vi "_Parse ACLR NR Limit Check Result.vi"(8 "error in (no error)":errorcluster, 10 "Input String":string, 11 "VISA resource name":refnum<visa-resource-name>) -> (0 "error out":errorcluster, 1 "ACLR Limit Check Results":T1, 2 "Reliability":i32, 3 "VISA resource name out":refnum<visa-resource-name>)   [LabVIEW 2020, in "Rohde&Schwarz CMWXP NR FR1 Measurement.lvlib"]
uses:
  <instrlib>/Rohde&Schwarz CMWXP NR FR1 Measurement/Rohde&Schwarz CMWXP NR FR1 Measurement.lvlib
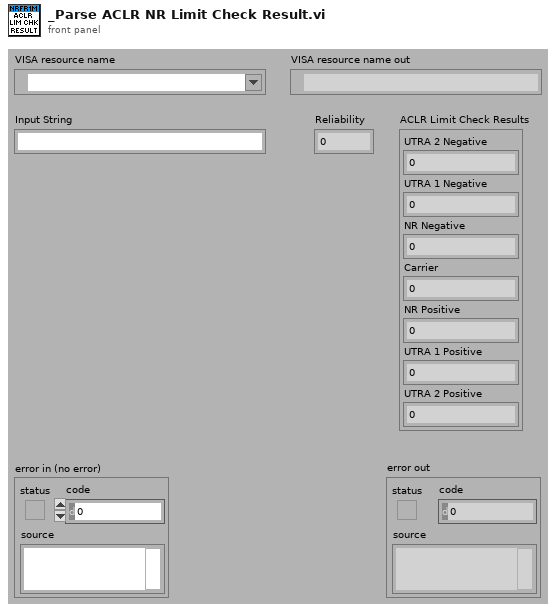
[diagram p1: front panel]
types:
  T1 = cluster{"UTRA 2 Negative":i32, "UTRA 1 Negative":i32, "NR Negative":i32, "Carrier":i32, "NR Positive":i32, "UTRA 1 Positive":i32, "UTRA 2 Positive":i32}
  T2 = cluster{"Limit Check Value":i32, "Limit Check Value":i32, "Limit Check Value":i32, "Limit Check Value":i32, "Limit Check Value":i32, "Limit Check Value":i32, "Limit Check Value":i32}
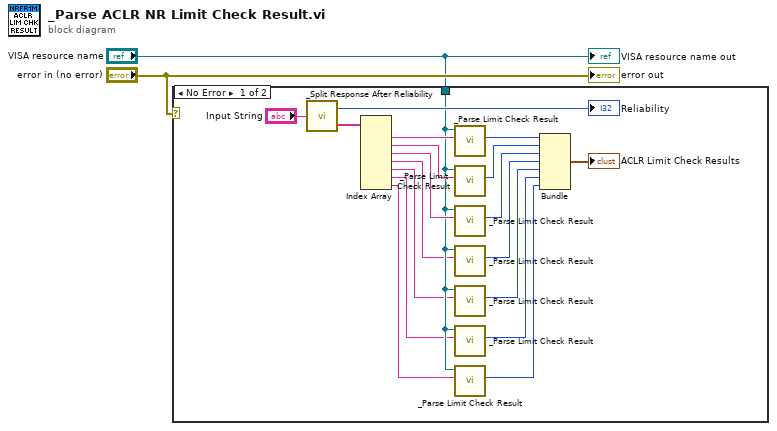
[diagram p0: block diagram]
diagram:
  n1 = case shown="No Error" "error in (no error)" {
    tunnel: "VISA resource name" -> [w11 _]
    frame No Error {
      n2 = call <instrlib>:"_Split Response After Reliability.vi"("Input String"="Input String") -> ("Response out"=w16:string[], "Reliability out"=→"Reliability":i32)
      n3 = Index Array(array=w16) -> (element #1=w15:string, element #2=w14:string, element #3=w13:string, element #4=w7:string, element #5=w8:string, element #6=w9:string, element #7=w10:string)  [unwired: 7 in]
      n4 = call <instrlib>:"_Parse Limit Check Result.vi"("String Value In"=w15, "VISA resource name"=w11) -> ("Limit Check Value"=w21:i32)  [unwired: 7 in, 2 out]
      n5 = call <instrlib>:"_Parse Limit Check Result.vi"("String Value In"=w14, "VISA resource name"=w11) -> ("Limit Check Value"=w20:i32)  [unwired: 7 in, 2 out]
      n6 = call <instrlib>:"_Parse Limit Check Result.vi"("String Value In"=w13, "VISA resource name"=w11) -> ("Limit Check Value"=w19:i32)  [unwired: 7 in, 2 out]
      n7 = call <instrlib>:"_Parse Limit Check Result.vi"("String Value In"=w7, "VISA resource name"=w11) -> ("Limit Check Value"=w6:i32)  [unwired: 7 in, 2 out]
      n8 = call <instrlib>:"_Parse Limit Check Result.vi"("String Value In"=w8, "VISA resource name"=w11) -> ("Limit Check Value"=w5:i32)  [unwired: 7 in, 2 out]
      n9 = call <instrlib>:"_Parse Limit Check Result.vi"("String Value In"=w9, "VISA resource name"=w11) -> ("Limit Check Value"=w4:i32)  [unwired: 7 in, 2 out]
      n10 = call <instrlib>:"_Parse Limit Check Result.vi"("String Value In"=w10, "VISA resource name"=w11) -> ("Limit Check Value"=w3:i32)  [unwired: 7 in, 2 out]
      n11 = Bundle("Limit Check Value"=w21, "Limit Check Value"=w20, "Limit Check Value"=w19, "Limit Check Value"=w6, "Limit Check Value"=w5, "Limit Check Value"=w4, "Limit Check Value"=w3) -> (→"ACLR Limit Check Results":T2)  [unwired: 1 in]
    }
    frame Error {
    }
  }
  "VISA resource name out" <- "VISA resource name"
  "error out" <- "error in (no error)"
